vi "Receiving Modulated Audio with SystemLink.vi"() -> ()   [LabVIEW 2019]
doc: "This application receives an audio modulated signal from the other target by communicating with a TCP protocol. The signal is then outputed through the EMONA Communications Board for its demodulation. After being demodulated, the signal is reproduced on the headphones and inputed once again to the application. Finally the application displays the message received through the Message Chart."
uses:
  <vilib>/Skyline/Tag/Shared/typedefs/DataType.ctl
  <vilib>/myRIO/Instrument Drivers/Onboard IO/AO Continuous/typedefs/AO Continuous Reference.ctl
  <vilib>/myRIO/Common/Instrument Driver Framework/Utilities/typedefs/myRIO Generic Hardware Reference.ctl
  <vilib>/myRIO/Common/Instrument Driver Framework/Utilities/typedefs/Hardware Version Enum.ctl
  <vilib>/myRIO/Common/Instrument Driver Framework/Utilities/typedefs/myRIO v1.0 Reference.ctl
  <vilib>/myRIO/Common/Instrument Driver Framework/Utilities/typedefs/Generic FPGA Reference.ctl
  <vilib>/myRIO/Common/Instrument Driver Framework/ELVIS III v1.0/AO Continuous/typedefs/AO Continuous Channels List.ctl
  <vilib>/myRIO/Common/Instrument Driver Framework/ELVIS III v1.0/AO Continuous/typedefs/ELVIS III v1.0 AO Continuous Channels Enum.ctl
  <vilib>/myRIO/Common/Instrument Driver Framework/ELVIS III v1.0/AO Continuous/typedefs/AO Continuous Channel Info.ctl
  <vilib>/userDefined/High Color/nirio_resource_hc.ctl
  <vilib>/myRIO/Instrument Drivers/Onboard IO/AI Block/typedefs/AI Block Reference.ctl
  <vilib>/myRIO/Common/Instrument Driver Framework/myRIO v1.0/AI Block/typedefs/AI Block Channels List.ctl
  <vilib>/myRIO/Common/Instrument Driver Framework/myRIO v1.0/AI Block/typedefs/AI Block Channels Enum.ctl
  <vilib>/myRIO/Common/Instrument Driver Framework/Utilities/typedefs/Analog Scaling Constants.ctl
  <vilib>/myRIO/Common/Instrument Driver Framework/ELVIS III v1.0/AO Continuous/vis/ELVIS III v1.1 Open AO (Continuous).vi
  <vilib>/myRIO/Common/Instrument Driver Framework/ELVIS III v1.0/AI Block/vis/ELVIS III v1.1 Open AI (N Samples).vi
  <vilib>/myRIO/Common/Instrument Driver Framework/Utilities/vis/Validate Channels.vi
  <vilib>/myRIO/Common/Instrument Driver Framework/ELVIS III v1.0/AO Continuous/vis/ELVIS III v1.0 Reserve AO Continuous.vi
  <vilib>/myRIO/Common/Instrument Driver Framework/ELVIS III v1.0/Resource Manager/vis/ELVIS III v1.0 Check For Different Banks.vi
  <vilib>/myRIO/Common/Instrument Driver Framework/ELVIS III v1.0/AI Block/vis/ELVIS III v1.0 AI Block Read.vi
  <vilib>/myRIO/Common/Instrument Driver Framework/ELVIS III v1.0/AO Continuous/vis/ELVIS III v1.1 Close AO Continuous.vi
  <vilib>/myRIO/Common/Instrument Driver Framework/ELVIS III v1.0/AI Block/vis/ELVIS III v1.0 Close AI Block.vi
  <vilib>/myRIO/Common/Instrument Driver Framework/myRIO v1.0/UART/vis/myRIO v1.0 Close UART.vi
  <vilib>/myRIO/Common/Instrument Driver Framework/ELVIS III v1.0/AO Continuous/vis/ELVIS III v1.0 Build MUX Configuration AO Continuous.vi
  <vilib>/myRIO/Common/Instrument Driver Framework/Utilities/vis/Sample Rate To Ticks.vi
  <vilib>/myRIO/Common/Instrument Driver Framework/ELVIS III v1.0/AO Continuous/vis/ELVIS III v1.0 Unreserve AO Continuous.vi
  <vilib>/myRIO/Common/Instrument Driver Framework/ELVIS III v1.0/AI Block/vis/ELVIS III v1.0 Unreserve AI Block.vi
  <vilib>/myRIO/Common/Instrument Driver Framework/ELVIS III v1.0/AI Block/vis/ELVIS III v1.0 Build MUX Configuration AI Block.vi
  <vilib>/Skyline/Configuration/Configuration HTTP_class/Open Configuration API Key.vi
  <vilib>/Skyline/Tag/Wrapper/Wrapper HTTP_class/Open Tag HTTP.vi
  <vilib>/Skyline/Tag/Wrapper/Wrapper_class/Write Tag (Boolean).vi
  <vilib>/Utility/VariantDataType/GetNumericInfo.vi
  <vilib>/Utility/error.llb/Error Cluster From Error Code.vi
  <vilib>/myRIO/Common/Instrument Driver Framework/ELVIS III v1.0/ELVIS III v1.1 Open.vi
  <vilib>/myRIO/Common/Instrument Driver Framework/ELVIS III v1.0/Resource Manager/vis/ELVIS III v1.0 Coerce AI Scaling.vi
  <vilib>/myRIO/Common/Instrument Driver Framework/ELVIS III v1.0/AI Block/vis/ELVIS III v1.0 Reserve AI Block.vi
  <vilib>/myRIO/Common/Instrument Driver Framework/ELVIS III v1.0/Resource Manager/vis/ELVIS III v1.0 Configure DMAs.vi
  <vilib>/myRIO/Common/Instrument Driver Framework/myRIO v1.0/myRIO v1.0 Close.vi
  <vilib>/myRIO/Common/Instrument Driver Framework/ELVIS III v1.0/Resource Manager/vis/ELVIS III v1.0 Reserve Channel List.vi
  <vilib>/myRIO/Common/Instrument Driver Framework/ELVIS III v1.0/AO Continuous/vis/ELVIS III v1.1 Stop AO Continuous.vi
  <vilib>/myRIO/Common/Instrument Driver Framework/ELVIS III v1.0/AO Continuous/vis/ELVIS III v1.0 AO Continuous Write.vi
  <vilib>/myRIO/Common/Instrument Driver Framework/ELVIS III v1.0/AO Continuous/vis/ELVIS III v1.1 Start AO Continuous.vi
  <vilib>/Skyline/Tag/Wrapper/Wrapper_class/Read Tag (Boolean).vi
  <vilib>/myRIO/Common/Instrument Driver Framework/myRIO v1.0/Resource Manager/vis/myRIO v1.0 Block Write Configuration.vi
  <vilib>/myRIO/Common/Instrument Driver Framework/ELVIS III v1.0/AI Block/vis/ELVIS III v1.0 AI Block Read Bank A.vi
  <vilib>/myRIO/Common/Instrument Driver Framework/ELVIS III v1.0/AI Block/vis/ELVIS III v1.0 AI Block Read Bank B.vi
  <vilib>/myRIO/Common/Instrument Driver Framework/ELVIS III v1.0/Resource Manager/vis/ELVIS III v1.0 Unreserve Channel List.vi
  <vilib>/Skyline/Tag/Wrapper/Wrapper_class/Close Tag (Single).vi
  <vilib>/myRIO/Common/Instrument Driver Framework/Utilities/vis/FPGA Ref Manager.vi
  <vilib>/myRIO/Common/Instrument Driver Framework/ELVIS III v1.0/ELVIS III v1.0 Reset FPGA.vi
  <vilib>/myRIO/Common/Instrument Driver Framework/myRIO v1.0/IRQ/vis/myRIO v1.0 IRQ Info FGV.vi
  <vilib>/myRIO/Common/Instrument Driver Framework/myRIO v1.0/IRQ/vis/myRIO v1.0 Timer IRQ Info FGV.vi
  <vilib>/myRIO/Common/Instrument Driver Framework/myRIO v1.0/IRQ/vis/myRIO v1.0 ISR Agent.vi
  <vilib>/myRIO/Instrument Drivers/Utilities/vis/Reset Index.vi
  <vilib>/myRIO/Common/Instrument Driver Framework/myRIO v1.0/Resource Manager/vis/myRIO v1.0 Block Write Resource Manager.vi
  <vilib>/Skyline/Tag/Wrapper/Wrapper_class/Write Tag (String).vi
  <vilib>/myRIO/Instrument Drivers/Onboard IO/AI Block/vis/myRIO AI N Samples Open.xnode
  <vilib>/myRIO/Instrument Drivers/Onboard IO/AO Continuous/vis/myRIO AO Continuous Open.xnode
  <vilib>/myRIO/Instrument Drivers/Utilities/Utilities.lvlib
  <vilib>/myRIO/Instrument Drivers/Onboard IO/AI Block/AI Block.lvlib
  <vilib>/myRIO/Instrument Drivers/Onboard IO/AO Continuous/AO Continuous.lvlib
  <vilib>/Skyline/Configuration/Configuration_class/NI Skyline Configuration.lvclass
  <vilib>/Skyline/Tag/Wrapper/Wrapper_class/NI Skyline Tag.lvclass
  <vilib>/Skyline/Tag/Shared/NI Skyline Tag.lvlib
  <vilib>/Skyline/Tag/Wrapper/Wrapper HTTP_class/NI Skyline Tag HTTP.lvclass
  <vilib>/Skyline/Configuration/Configuration HTTP_class/NI Skyline Configuration HTTP.lvclass
panel:
  out "Demodulator":string caption="Demodulator IP Address"
  out "Message":dbl[](graph)
  out "Signal":dbl[](graph) caption="Modulated Signal"
  out "Error Out":errorcluster
  in  "Stop":bool
  # "Receiving and Demodulating Audio"
  # "Explanation:\nThis application receives an audio modulated signal from the other target by communicating with a TCP protocol. The signal is then outputed through the EMONA Communications Board for its demodulation. After being demodulated, the signal is reproduced on the headphones and inputed once again to the application. Finally the application displays the message received through the Message Chart.\n \nThe audio from the target might sound lightly distortioned because of the modulation and demodulation process that was applied to the signal.\n \nInstructions:\n •  Make sure that you have uploaded at least one audio file to the Modulating target for its reproduction (use the Uploading Audio Files VI to do this).\n • Deploy the matching VIs (Sending and Receiving) to each target.\n • Enter the text from the indicator below into the Demodulator IP Address control from the Sending Modulated Audio.vi.\n • Run this VI again and afterwards run the other VI.\n • Try changing between songs and hearing the audio from both targets.\n • If you are not going to use any of the VIs from this project anymore, run the Remove Audio Files VI on the other target."
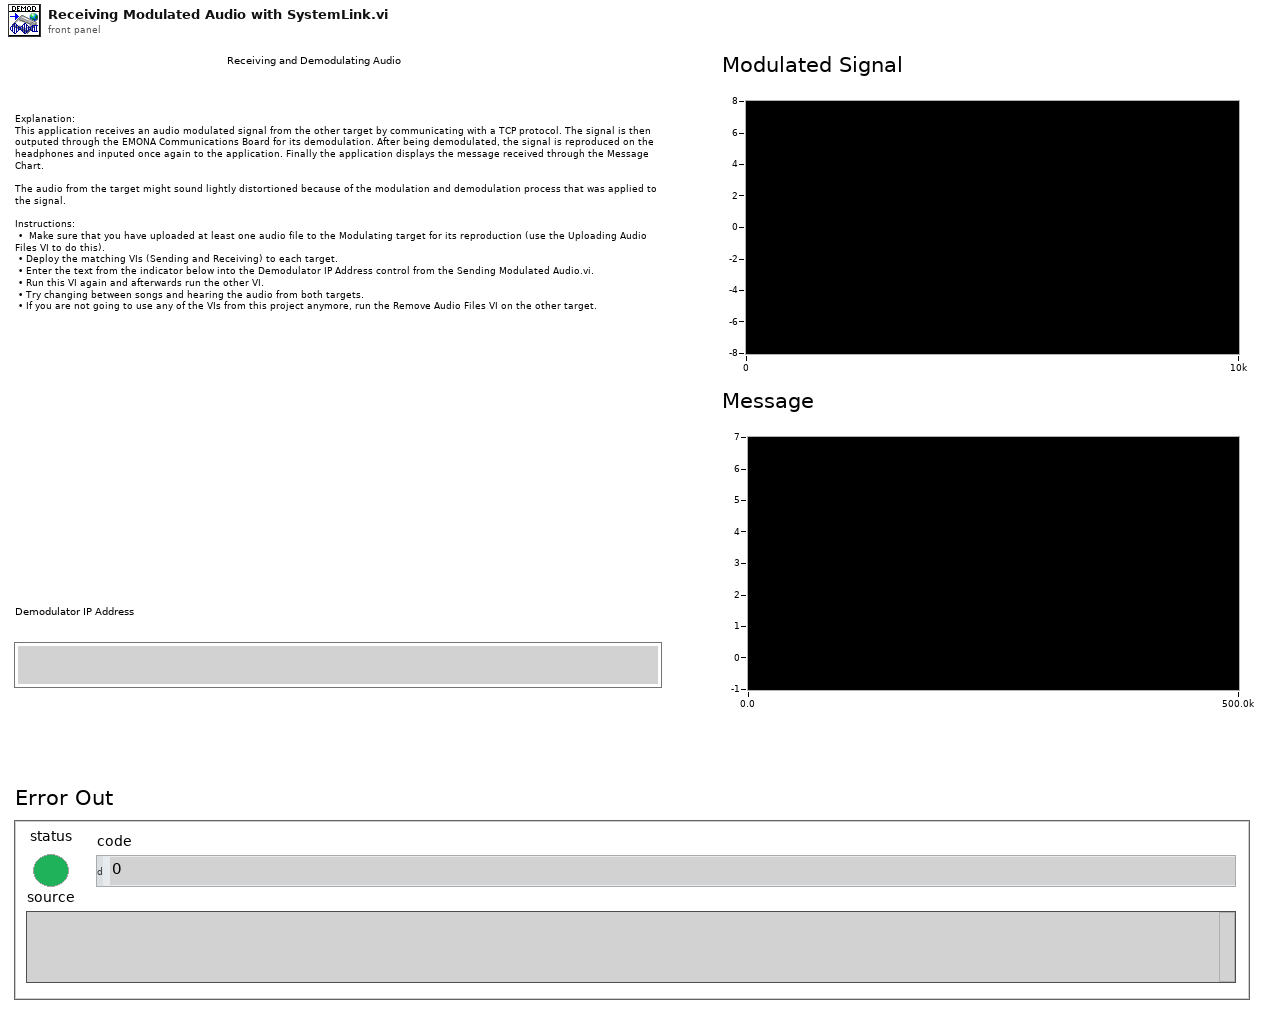
[diagram p1: front panel]
types:
  T1 = typedef "NI Skyline Tag.lvlib/DataType.ctl" = enum32{"Double", "I32", "String", "Boolean", "U64", "Timestamp"}
  T2 = typedef "AO Continuous.lvlib/AO Continuous Reference.ctl" = cluster{"myRIO Reference":T3, "AO (Continuous) Channels List":T7, "Channel Info":T9}
  T3 = typedef "myRIO Generic Hardware Reference.ctl" = cluster{"myRIO Model":T4, "myRIO Hardware Reference":T5}
  T4 = typedef "Hardware Version Enum.ctl" = enum16{"Unknown", "myRIO-1900", "myRIO-1950", "roboRIO", "NI ELVIS RIO CM", "ELVIS III"}
  T5 = typedef "myRIO v1.0 Reference.ctl" = cluster{"Generic FPGA Reference":T6, "Allow multiple opens":bool}
  T6 = typedef "Generic FPGA Reference.ctl" = refnum<k20>
  T7 = typedef "AO Continuous Channels List.ctl" = T8[]
  T8 = typedef "ELVIS III v1.0 AO Continuous Channels Enum.ctl" = enum16{"Not Connected", "A/AO0 (Continuous)", "A/AO1 (Continuous)", "B/AO0 (Continuous)", "B/AO1 (Continuous)"}
  T9 = typedef "AO Continuous Channel Info.ctl" = cluster{"Channel Bitmask":u8[], "Channel Index":i32[], "Channel Number":u8}
  T10 = typedef "AI Block.lvlib/AI Block Reference.ctl" = cluster{"myRIO Reference":T3, "AI (N Samples) Channels List":T11, "AI (N Samples) Scaling Constants List":T13[]}
  T11 = typedef "AI Block Channels List.ctl" = T12[]
  T12 = typedef "AI Block Channels Enum.ctl" = enum16{"Not Connected", "A/AI0 (N Samples)", "A/AI1 (N Samples)", "A/AI2 (N Samples)", "A/AI3 (N Samples)", "A/AI4 (N Samples)", "A/AI5 (N Samples)", "A/AI6 (N Samples)", "A/AI7 (N Samples)", "A/AI0 (DIFF N Samples)", "A/AI1 (DIFF N Samples)", "A/AI2 (DIFF N Samples)", "A/AI3 (DIFF N Samples)", "B/AI0 (N Samples)", "B/AI1 (N Samples)", "B/AI2 (N Samples)", "B/AI3 (N Samples)", "B/AI4 (N Samples)", "B/AI5 (N Samples)", "B/AI6 (N Samples)", "B/AI7 (N Samples)", "B/AI0 (DIFF N Samples)", "B/AI1 (DIFF N Samples)", "B/AI2 (DIFF N Samples)", "B/AI3 (DIFF N Samples)"}
  T13 = typedef "Analog Scaling Constants.ctl" = cluster{"LSB Weight (Volts)":dbl, "Offset (Volts)":dbl, "Signed?":bool}
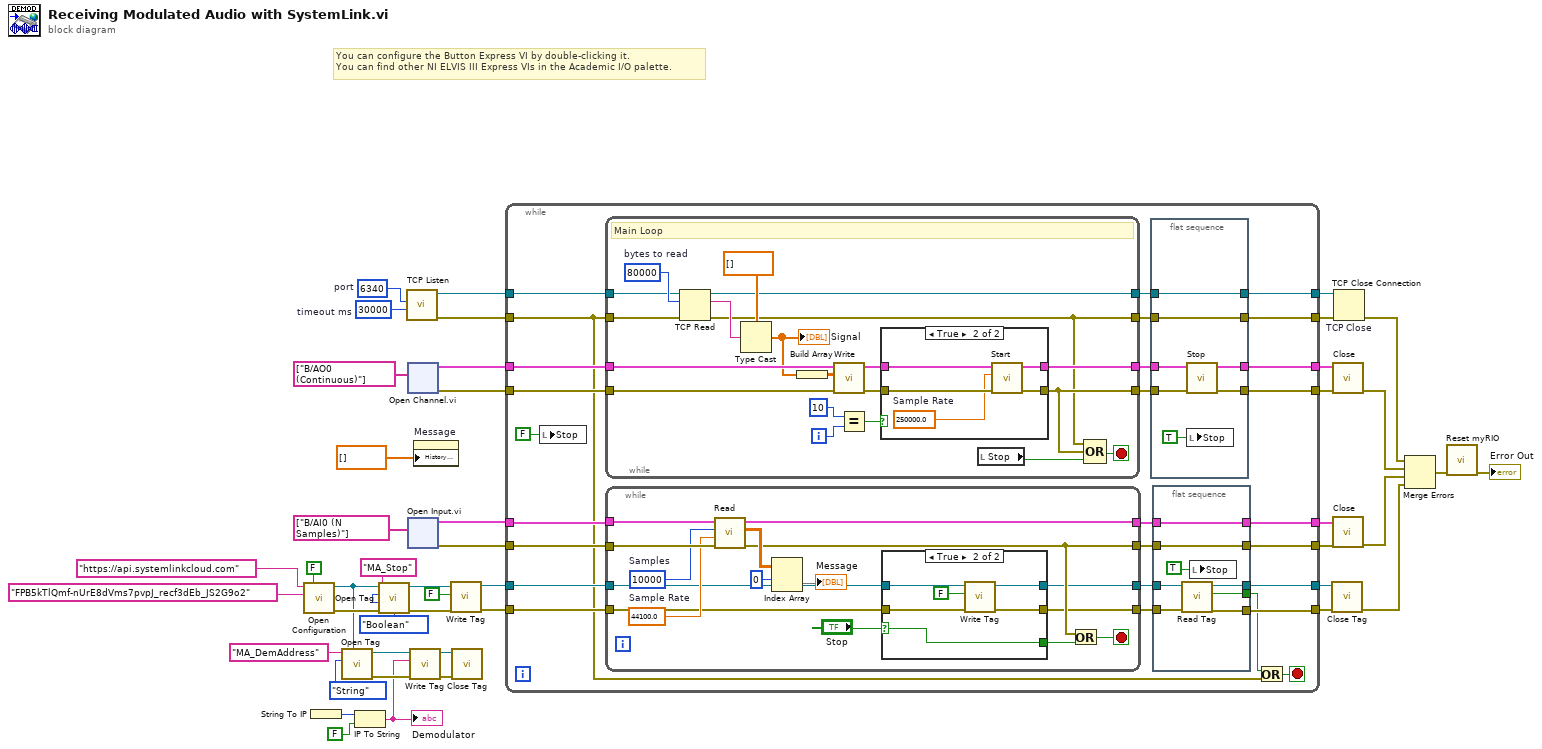
[diagram p0: block diagram]
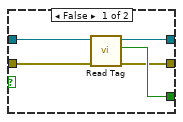
[diagram p2: hidden frame]
diagram:
  w10 = 30000  # timeout ms
  w9 = u16 6340  # port
  # "You can configure the Button Express VI by double-clicking it.\nYou can find other NI ELVIS III Express VIs in the Academic I/O palette."
  n1 = call-poly <vilib>:"Open Configuration.vi"("verify server?"=FALSE, "api key"="FPB5kTlQmf-nUrE8dVms7pvpJ_recf3dEb_JS2G9o2", "server url"="https://api.systemlinkcloud.com") -> ("error out"=w29:errorcluster, "HTTP configuration out"=w24:refnum<class "NI Skyline Configuration HTTP.lvclass">)  [unwired: 7 in]
  n2 = String To IP() -> (0:w32:u32)  [unwired: 1 in]
  n3 = call-poly <vilib>:"Open Tag.vi"("configuration"=w24, "Data Type"=DataType."String", "path"="MA_DemAddress") -> ("error out"=w27:errorcluster, "tag out"=w28:refnum<class "NI Skyline Tag.lvclass">)  [unwired: 7 in]
  n4 = IP To String(1:FALSE ("dot notation? (F)"), 2:w32) -> (0:w1:string)
  "Demodulator" <- w1
  n5 = call-poly <vilib>:"Open Tag.vi"("configuration"=w24, "error in (no error)"=w29, "Data Type"=DataType."Boolean", "path"="MA_Stop") -> ("error out"=w30:errorcluster, "tag out"=w31:refnum<class "NI Skyline Tag.lvclass">)  [unwired: 6 in]
  n6 = call <vilib>:"TCP Listen.vi"("timeout ms (wait forever: -1)"=w10, "port"=w9) -> ("error out"=w7:errorcluster, "connection ID"=w8:refnum<k5>)  [unwired: 5 in, 3 out]
  n7 = xnode "Open Channel.vi"("Channel Names"=tag[] ["B/AO0 (Continuous)"]) -> ("error out"=w41:errorcluster, "AO (Continuous) Ref Out"=w42:T2)  [unwired: 1 in]
  n8 = xnode "Open Input.vi"("Channel Names"=tag[] ["B/AI0 (N Samples)"]) -> ("error out"=w46:errorcluster, "AI (N Samples) Ref Out"=w45:T10)  [unwired: 4 in]
  n9 = call-poly <vilib>:"Write Tag.vi"("error in (no error)"=w27, "value"=w1, "tag in"=w28) -> ("error out"=w25:errorcluster, "tag out"=w26:refnum<class "NI Skyline Tag.lvclass">)  [unwired: 7 in]
  n10 = property on="Message" class="WFChart (strict)"("History Data"=dbl[] []) -> ()  [unwired: 2 in, 2 out]
  n11 = call-poly <vilib>:"Write Tag.vi"("error in (no error)"=w30, "value"=FALSE, "tag in"=w31) -> ("error out"=w37:errorcluster, "tag out"=w38:refnum<class "NI Skyline Tag.lvclass">)  [unwired: 7 in]
  n12 = call-poly <vilib>:"Close Tag.vi"("error in (no error)"=w25, "tag in"=w26) -> ()  [unwired: 9 in, 1 out]
  n13 = while {
    tunnel: w37 -> [w65]
    tunnel: [w63] -> w35
    tunnel: w38 -> [w66]
    tunnel: [w64] -> w36
    tunnel: w46 -> [w73]
    tunnel: [w71] -> w44
    tunnel: w45 -> [w72]
    tunnel: [w70] -> w43
    tunnel: w41 -> [w48]
    tunnel: [w68] -> w40
    tunnel: w42 -> [w69]
    tunnel: [w67] -> w39
    tunnel: [w53] -> w5
    tunnel: w8 -> [w52]
    tunnel: w7 -> [w47]
    tunnel: [w51] -> w6
    stop <- w49 stop-if-true
    n14 = local write "Stop"(FALSE ("Stop")) -> ()
    n15 = while {
      tunnel: w48 -> [w131]
      tunnel: [w125] -> w61
      tunnel: w69 -> [w132]
      tunnel: [w130] -> w62
      tunnel: w52 -> [w120]
      tunnel: w47 -> [w119]
      tunnel: [w122] -> w58
      tunnel: [w118] -> w57
      i -> [w127]
      stop <- w135 stop-if-true
      w121 = 80000  # bytes to read
      # "Main Loop"
      n16 = TCP Read(connection ID=w120, bytes to read=w121, error in (no error)=w119) -> (connection ID out=w122:refnum<k5>, data out=w123:string, error out=w118:errorcluster)  [unwired: 2 in]
      n17 = Type Cast(type=dbl[] [] ("chart"), x=w123) -> (*(type *) &x=w116:dbl[])
      "Signal" <- w116
      n18 = Build Array(w116) -> (w129:dbl[][])
      n19 = call <vilib>:"Write.vi"("error in (no error)"=w131, "Data To Write"=w129, "AO (Continuous) Ref In"=w132) -> ("error out"=w133:errorcluster, "AO (Continuous) Ref Out"=w134:T2)  [unwired: 7 in]
      n20 = Equal?(x=10, y=w127) -> (x = y?=w128:bool)
      n21 = case shown="True" w128 {
        tunnel: w134 -> [w137 w142]
        tunnel: w133 -> [w136 w141]
        tunnel: [w137 w140] -> w130
        tunnel: [w136 w139] -> w125
        frame False {
        }
        frame True {
          w138 = 250000.0  # Sample Rate
          n22 = call <vilib>:"Start.vi"("error in (no error)"=w141, "Sample Rate"=w138, "AO (Continuous) Ref In"=w142) -> ("error out"=w139:errorcluster, "AO (Continuous) Ref Out"=w140:T2)  [unwired: 7 in]
        }
      }
      n23 = local read "Stop"() -> (w117:bool)
      n24 = Compound Arithmetic op=OR(w118, w125, w117) -> (w135:bool)
    }
    n25 = while {
      tunnel: w72 -> [w104]
      tunnel: [w101] -> w60
      tunnel: w73 -> [w103]
      tunnel: [w96] -> w59
      tunnel: w66 -> [w95]
      tunnel: w65 -> [w94]
      tunnel: [w93] -> w56
      tunnel: [w92] -> w55
      stop <- w102 stop-if-true
      w97 = u32 10000  # Samples
      w98 = 44100.0  # Sample Rate
      n26 = call <vilib>:"Read.vi"("error in (no error)"=w103, "Sample Rate [Hz]"=w98, "Number of Samples"=w97, "AI (N Samples) Ref In"=w104) -> ("error out"=w96:errorcluster, "Values"=w100:dbl[][], "AI (N Samples) Ref Out"=w101:T10)  [unwired: 5 in]
      n27 = Index Array(array=w100, index (row)=0) -> (element=→"Message":dbl[])  [unwired: 1 in]
      n28 = case shown="True" "Stop" {
        selector: "Stop" -> [_ w113]
        tunnel: w94 -> [w108 w115]
        tunnel: w95 -> [w109 w114]
        tunnel: [w107 w113] -> w91
        tunnel: [w106 w112] -> w93
        tunnel: [w105 w111] -> w92
        frame False {
          n29 = call-poly <vilib>:"Read Tag.vi"("error in (no error)"=w108, "tag in"=w109) -> ("error out"=w105:errorcluster, "value"=w107:bool, "tag out"=w106:refnum<class "NI Skyline Tag.lvclass">)  [unwired: 5 in, 2 out]
        }
        frame True {
          n30 = call-poly <vilib>:"Write Tag.vi"("error in (no error)"=w115, "value"=FALSE, "tag in"=w114) -> ("error out"=w111:errorcluster, "tag out"=w112:refnum<class "NI Skyline Tag.lvclass">)  [unwired: 7 in]
        }
      }
      n31 = Or(x=w96, y=w91) -> (x .or. y?=w102:bool)
    }
    n32 = flat-sequence {
      tunnel: w62 -> [w85]
      tunnel: w61 -> [w84]
      tunnel: [w87] -> w68
      tunnel: [w86] -> w67
      tunnel: w58 -> [w83]
      tunnel: w57 -> [w82]
      tunnel: [w82] -> w53
      tunnel: [w83] -> w51
      frame #0 {
        n33 = call <vilib>:"Stop.vi"("error in (no error)"=w84, "AO (Continuous) Ref In"=w85) -> ("error out"=w87:errorcluster, "AO (Continuous) Ref Out"=w86:T2)  [unwired: 8 in]
        n34 = local write "Stop"(TRUE ("Stop")) -> ()
      }
    }
    n35 = flat-sequence {
      tunnel: w60 -> [w81]
      tunnel: [w81] -> w70
      tunnel: w59 -> [w80]
      tunnel: [w80] -> w71
      tunnel: w56 -> [w78]
      tunnel: [w75] -> w64
      tunnel: [w77] -> w63
      tunnel: w55 -> [w76]
      tunnel: [w74] -> w50
      frame #0 {
        n36 = call-poly <vilib>:"Read Tag.vi"("error in (no error)"=w76, "tag in"=w78) -> ("error out"=w77:errorcluster, "value"=w74:bool, "tag out"=w75:refnum<class "NI Skyline Tag.lvclass">)  [unwired: 5 in, 2 out]
        n37 = local write "Stop"(TRUE ("Stop")) -> ()
      }
    }
    n38 = Or(x=w50, y=w47) -> (x .or. y?=w49:bool)
  }
  n39 = call-poly <vilib>:"Close Tag.vi"("error in (no error)"=w35, "tag in"=w36) -> ("error out"=w11:errorcluster)  [unwired: 9 in]
  n40 = call <vilib>:"Close.vi"("error in (no error)"=w40, "AO (Continuous) Ref In"=w39) -> ("error out"=w13:errorcluster)  [unwired: 9 in]
  n41 = call <vilib>:"Close.vi"("error in (no error)"=w44, "AI (N Samples) Ref In"=w43) -> ("error out"=w12:errorcluster)  [unwired: 9 in]
  n42 = TCP Close Connection "TCP Close"(connection ID=w6, error in (no error)=w5) -> (error out=w4:errorcluster)  [unwired: 1 in, 1 out]
  n43 = Merge Errors(w4, w13, w12, w11) -> (w14:errorcluster)
  n44 = call <vilib>:"Reset myRIO.vi"("error in (no error)"=w14) -> ("error out"=→"Error Out":errorcluster)  [unwired: 10 in]
